vi "Teleop.vi"(10 "Match Info":T1={"Autonomous Elapsed Seconds"=0.0, "TeleOp Elapsed Seconds"=0.0, "Disabled Elapsed Seconds"=0.0, "Visited Autonomous"=FALSE, "Visited TeleOp"=FALSE, "Visited Disabled"=FALSE, "Autonomous Settings"={"Autonomous Style"=enum."Independent", "VI Refnum"=refnum}}, 11 "Call Context":T2) -> ()   [LabVIEW 2016]
doc: "This VI is called for each TeleOp packet received from the DS where the robot is not disabled. It is often used to read from the joysticks and update I/O or to update setpoints for timed control loops. It should complete and return within 20 milliseconds or it may miss DS packets."
uses:
  <vilib>/Rock Robotics/WPI/DriverStation/WPI_DriverStationDerivedRobotMode.ctl
  <vilib>/Rock Robotics/WPI/DriverStation/WPI_DriverStationMatch Info.ctl
  <vilib>/Rock Robotics/WPI/Utilities/WPI_GetSetVariantRefNum.vi
  Extra/Global_Var_Drive.vi
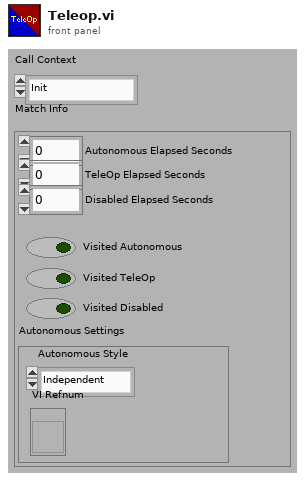
[diagram p1: front panel]
types:
  T1 = typedef "WPI_DriverStationMatch Info.ctl" = cluster{"Autonomous Elapsed Seconds":dbl, "TeleOp Elapsed Seconds":dbl, "Disabled Elapsed Seconds":dbl, "Visited Autonomous":bool, "Visited TeleOp":bool, "Visited Disabled":bool, "Autonomous Settings":cluster{"Autonomous Style":enum16{"Iterative", "Independent"}, "VI Refnum":refnum<vi>}}
  T2 = typedef "WPI_DriverStationDerivedRobotMode.ctl" = enum16{"Init", "Execute", "Stop"}
  T3 = typedef "WPI_JoystickDevRef.ctl" = cluster{"Device":T4}
  T4 = typedef "WPI_JoystickDeviceEnum.ctl" = enum16{"USB 0", "USB 1", "USB 2", "USB 3", "USB 4", "USB 5"}
  T5 = cluster{"Left_Trigger":dbl, "Right_Trigger ":dbl, "Left_X":dbl, "Left_Y":dbl, "Right_X":dbl, "Right_Y":dbl}
  T6 = cluster{"A":bool, "B":bool, "X":bool, " Y":bool, "LB":bool, " RB":bool, "Left_Thumb_Button":bool, "Right_Thumb_Button":bool, "Back":bool, "Start":bool}
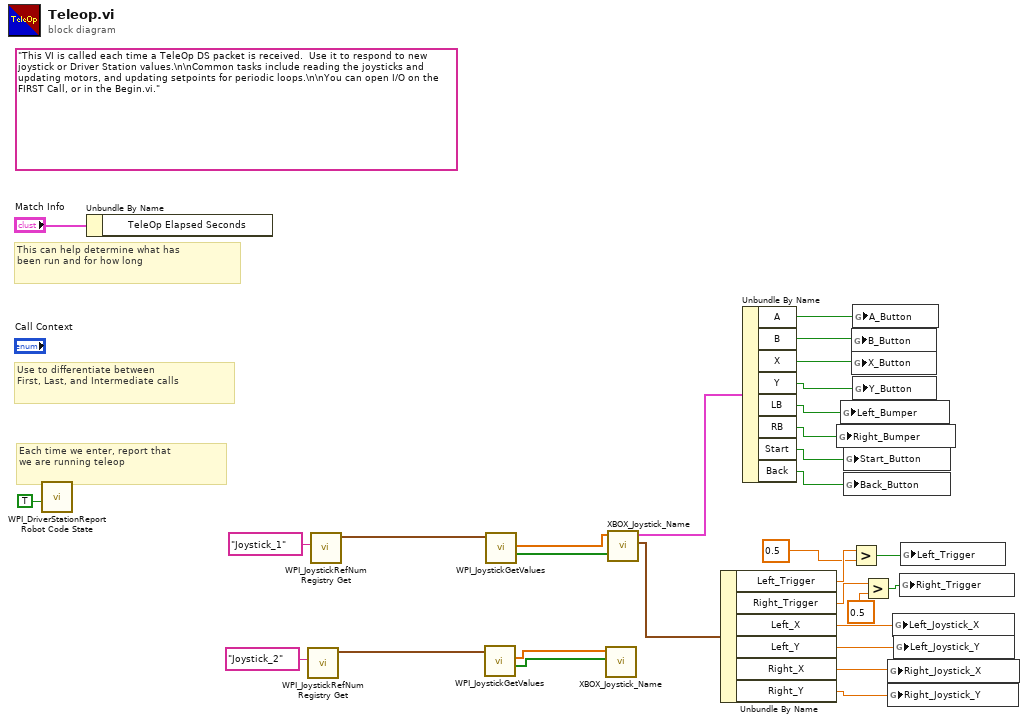
[diagram p0: block diagram]
diagram:
  (unwired) "This VI is called each time a TeleOp DS packet is received.  Use it to respond to new joystick or Driver Station values.\n\nCommon tasks include reading the joysticks and updating motors, and updating setpoints for periodic loops.\n\nYou can open I/O on the FIRST Call, or in the Begin.vi."
  # "Each time we enter, report that\nwe are running teleop"
  # "Use to differentiate between\nFirst, Last, and Intermediate calls"
  # "This can help determine what has\nbeen run and for how long"
  n1 = call <vilib>:"WPI_DriverStationReport Robot Code State.vi"("TeleOp"=TRUE ("Autonomous")) -> ()  [unwired: 10 in, 1 out]
  n2 = Unbundle By Name("Match Info") -> ()  [unwired: 1 out]
  n3 = call <vilib>:"WPI_JoystickRefNum Registry Get.vi"("refnum name"="Joystick_2") -> ("JoystickDevRef"=w25:T3)  [unwired: 9 in, 1 out]
  n4 = call <vilib>:"WPI_JoystickRefNum Registry Get.vi"("refnum name"="Joystick_1") -> ("JoystickDevRef"=w26:T3)  [unwired: 9 in, 1 out]
  n5 = call <vilib>:"WPI_JoystickGetValues.vi"("JoystickDevRef"=w25) -> ("Buttons"=w21:bool[], "Axes"=w22:dbl[])  [unwired: 6 in, 3 out]
  n6 = call <vilib>:"WPI_JoystickGetValues.vi"("JoystickDevRef"=w26) -> ("Buttons"=w24:bool[], "Axes"=w23:dbl[])  [unwired: 6 in, 3 out]
  n7 = call "XBOX_Joystick_Name.vi"("Buttons"=w21, "Axes"=w22) -> ()  [unwired: 8 in, 2 out]
  n8 = call "XBOX_Joystick_Name.vi"("Buttons"=w24, "Axes"=w23) -> ("Named_Joystick"=w19:T5, "Named_Buttons"=w20:T6)  [unwired: 8 in]
  n9 = Unbundle By Name(w19) -> ("Left_Trigger"=w14:dbl, "Right_Trigger"=w11:dbl, "Left_X"=w18:dbl, "Left_Y"=w17:dbl, "Right_X"=w16:dbl, "Right_Y"=w15:dbl)
  n10 = Unbundle By Name(w20) -> ("A"=w8:bool, "B"=w7:bool, "X"=w6:bool, "Y"=w5:bool, "LB"=w4:bool, "RB"=w3:bool, "Start"=w2:bool, "Back"=w1:bool)
  n11 = global write "Global_Var_Drive.vi" "Right_Bumper"(w3) -> ()
  n12 = global write "Global_Var_Drive.vi" "Left_Bumper"(w4) -> ()
  n13 = global write "Global_Var_Drive.vi" "Start_Button"(w2) -> ()
  n14 = global write "Global_Var_Drive.vi" "Back_Button"(w1) -> ()
  n15 = Greater?(x=w14, y=0.5) -> (0:w12:bool)
  n16 = global write "Global_Var_Drive.vi" "B_Button"(w7) -> ()
  n17 = global write "Global_Var_Drive.vi" "X_Button"(w6) -> ()
  n18 = global write "Global_Var_Drive.vi" "A_Button"(w8) -> ()
  n19 = global write "Global_Var_Drive.vi" "Y_Button"(w5) -> ()
  n20 = Greater?(x=w11, y=0.5) -> (0:w9:bool)
  n21 = global write "Global_Var_Drive.vi" "Right_Joystick_X"(w16) -> ()
  n22 = global write "Global_Var_Drive.vi" "Right_Joystick_Y"(w15) -> ()
  n23 = global write "Global_Var_Drive.vi" "Left_Joystick_X"(w18) -> ()
  n24 = global write "Global_Var_Drive.vi" "Left_Joystick_Y"(w17) -> ()
  n25 = global write "Global_Var_Drive.vi" "Right_Trigger"(w9) -> ()
  n26 = global write "Global_Var_Drive.vi" "Left_Trigger"(w12) -> ()
